vi "CAL_GCP_L_power.vi"(8 "L_power_raw":sgl, 9 "출력 클러스터 2":T1, 10 "B_ACC":sgl, 11 "L_ROLL":sgl) -> (0 "L_Period":sgl, 1 "L_GCP":sgl, 2 "L_Ctrl_Start":bool, 3 "L_NUM":u32, 4 "L_Run_OK":bool, 5 "출력 클러스터":T1)   [LabVIEW 2019]
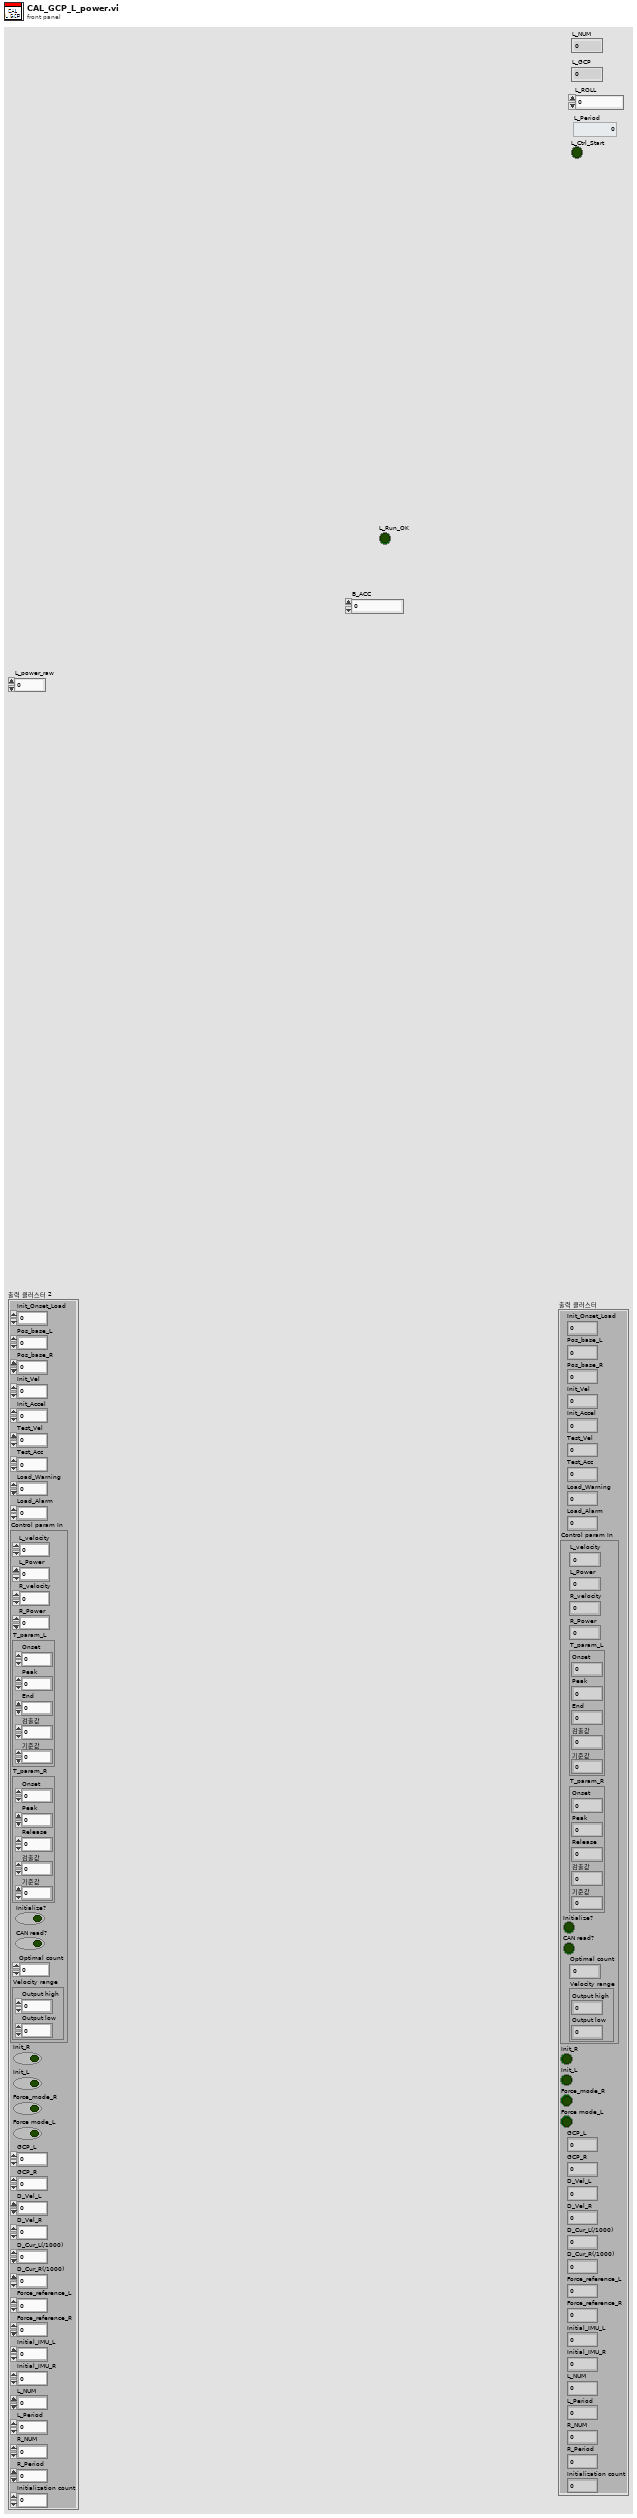
[diagram p1: front panel]
types:
  T1 = cluster{"Init_Onset_Load":sgl, "Pos_base_L":sgl, "Pos_base_R":sgl, "Init_Vel":i32, "Init_Accel":u32, "Test_Vel":i32, "Test_Acc":u32, "Load_Warning":sgl, "Load_Alarm":sgl, "Control param In":cluster{"L_velocity":u32, "L_Power":sgl, "R_velocity":u32, "R_Power":sgl, "T_param_L":cluster{"Onset":sgl, "Peak":sgl, "End":sgl, "검출값":sgl, "기준값":sgl}, "T_param_R":cluster{"Onset":sgl, "Peak":sgl, "Release":sgl, "검출값":sgl, "기준값":sgl}, "Initialize?":bool, "CAN read?":bool, "Optimal count":i32, "Velocity range":cluster{"Output high":dbl, "Output low":dbl}}, "Init_R":bool, "Init_L":bool, "Force_mode_R":bool, "Force mode_L":bool, "GCP_L":sgl, "GCP_R":sgl, "D_Vel_L":sgl, "D_Vel_R":sgl, "D_Cur_L(/1000)":sgl, "D_Cur_R(/1000)":sgl, "Force_reference_L":sgl, "Force_reference_R":sgl, "Initial_IMU_L":sgl, "Initial_IMU_R":sgl, "L_NUM":u32, "L_Period":i16, "R_NUM":u32, "R_Period":i16, "Initialization count":i32}
  T2 = enum16{"Init", "HF", "Cross", "HE", "Cross_E", "Init_F"}
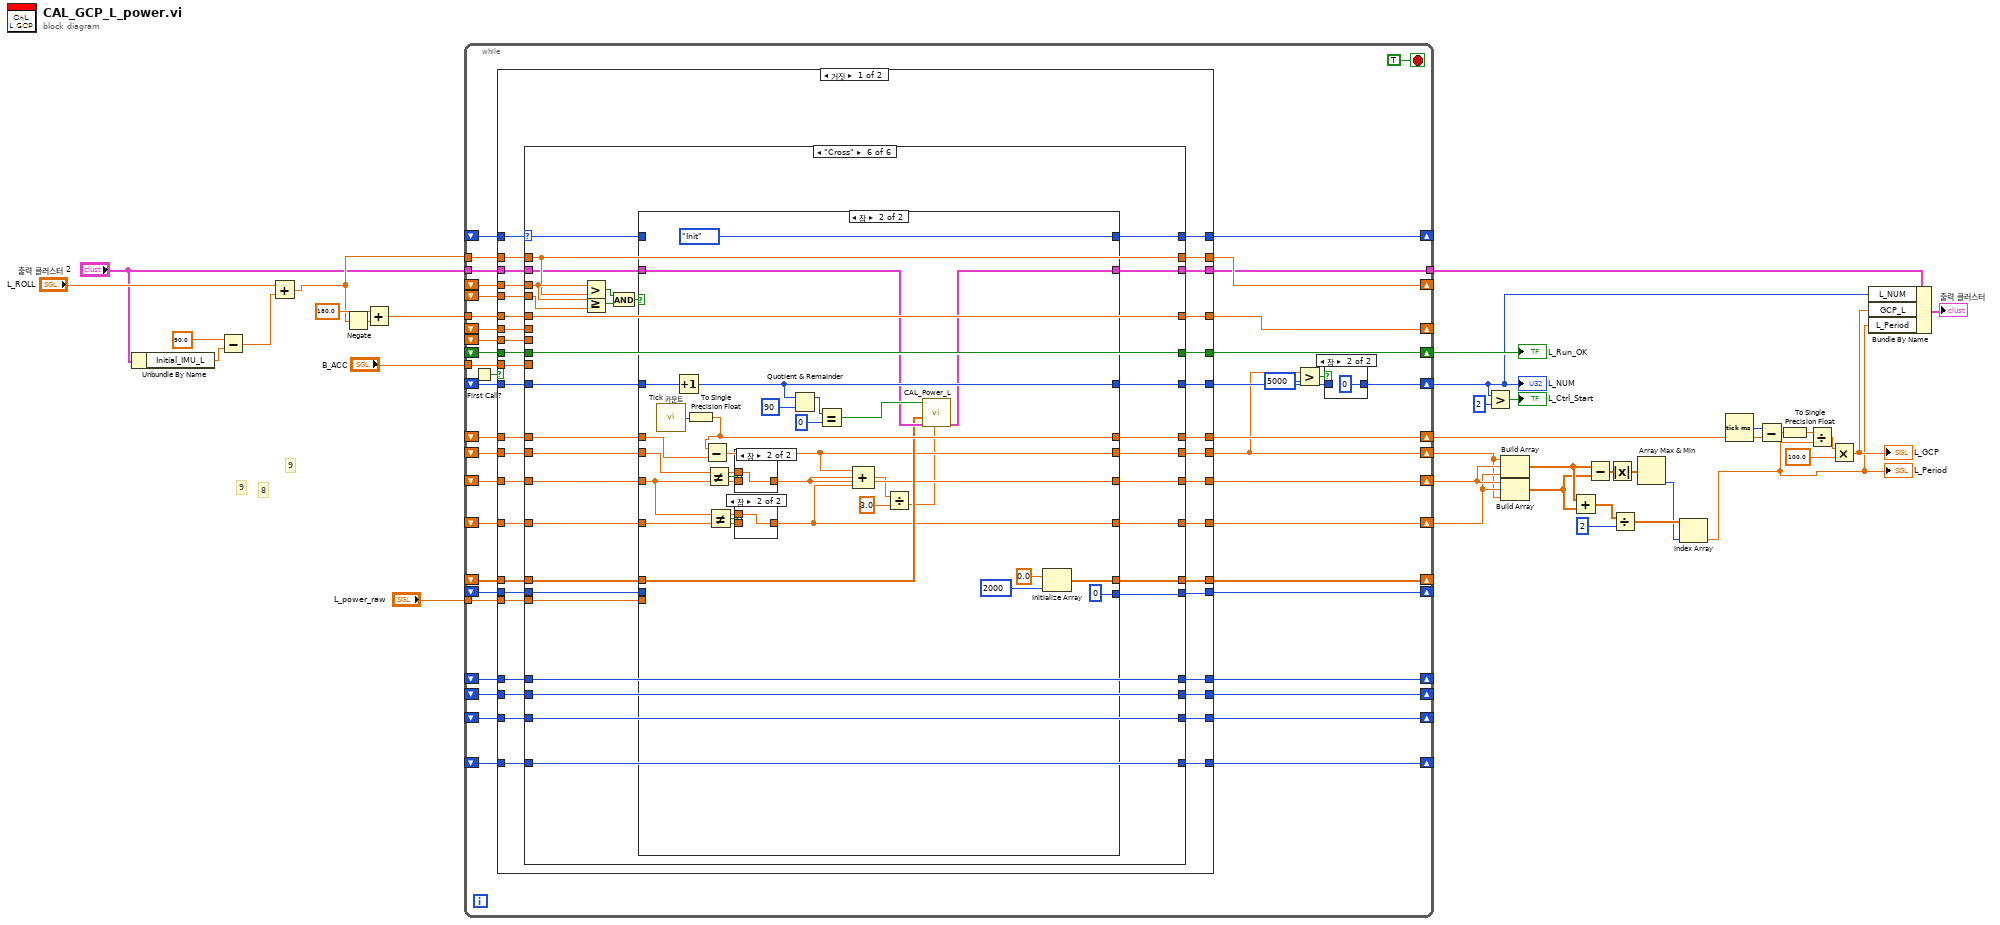
[diagram p0: block diagram]
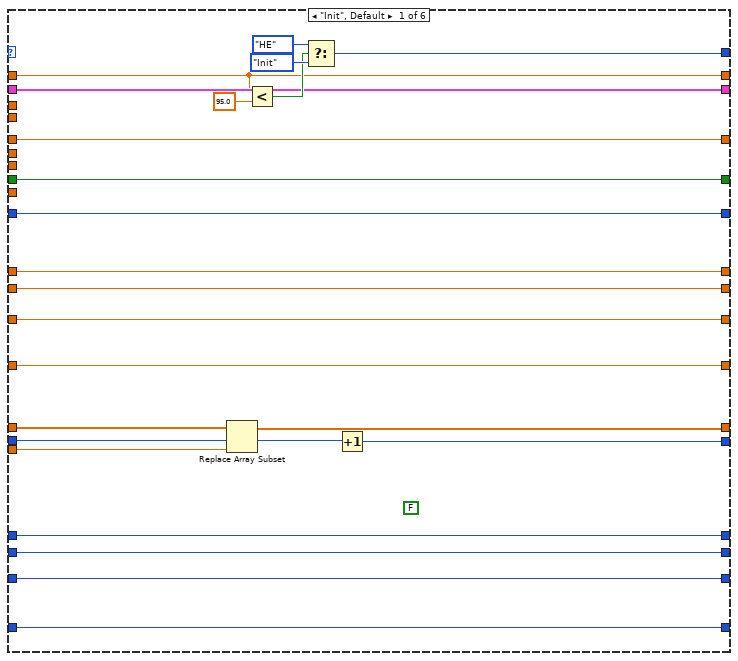
[diagram p2: hidden frame]
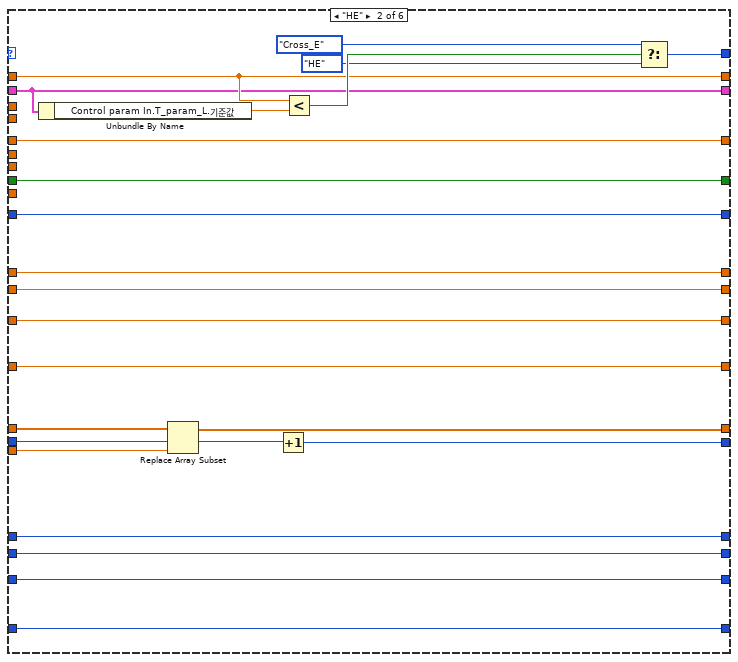
[diagram p3: hidden frame]
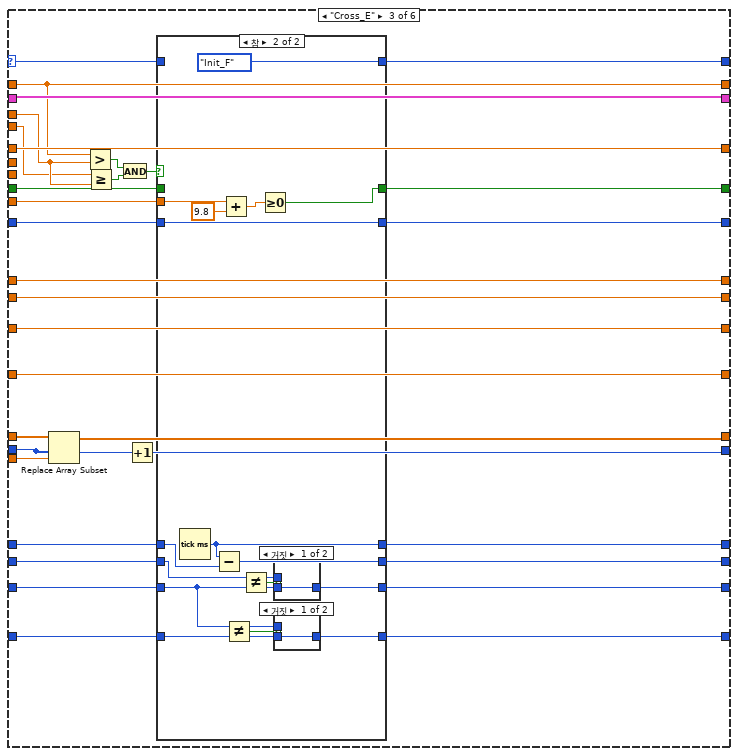
[diagram p4: hidden frame]
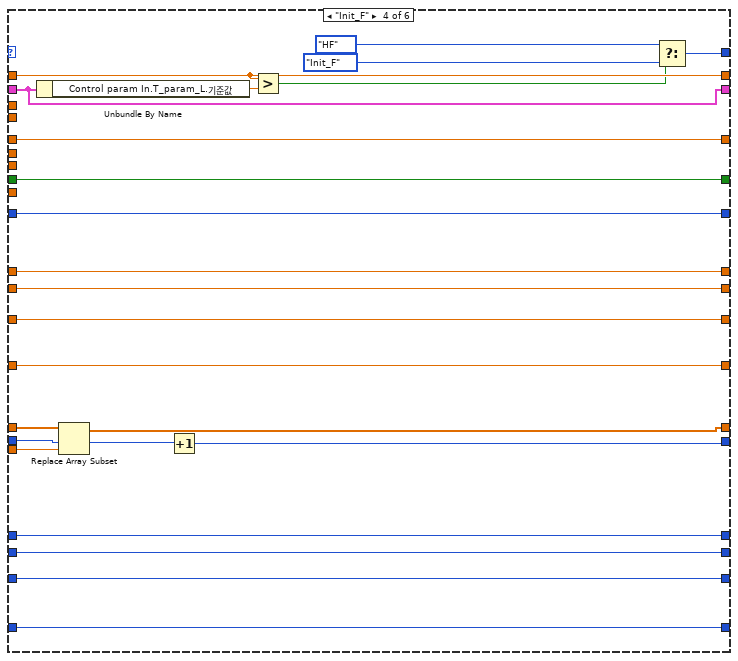
[diagram p8: hidden frame]
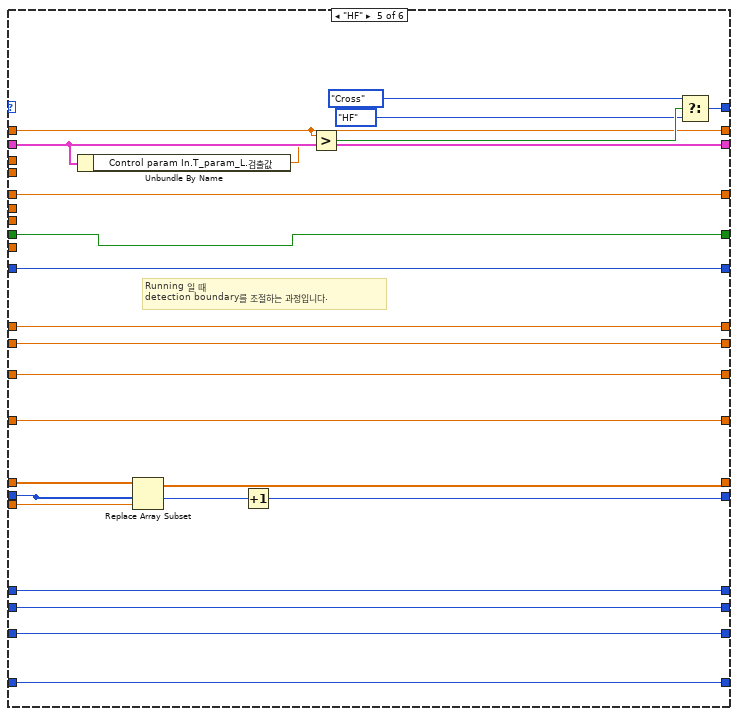
[diagram p9: hidden frame]
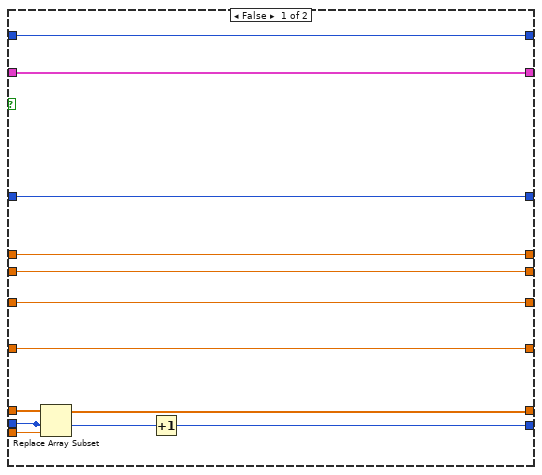
[diagram p10: hidden frame]
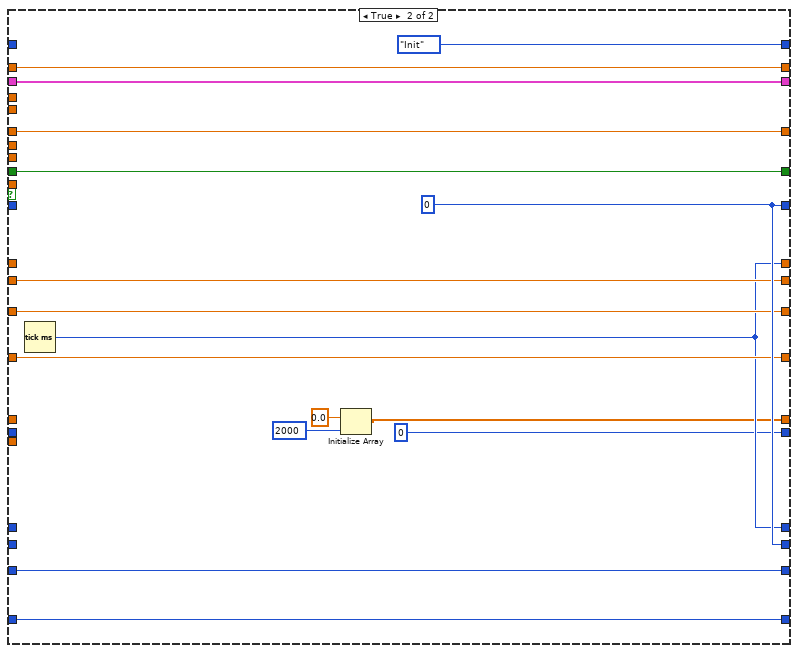
[diagram p13: hidden frame]
diagram:
  # "9"
  # "8"
  # "9"
  n1 = Unbundle By Name("출력 클러스터 2") -> ("Initial_IMU_L"=w5:sgl)
  n2 = Subtract(x=sgl 90.0 ("y"), y=w5) -> (x-y=w1:sgl)
  n3 = Add(x="L_ROLL", y=w1) -> (x+y=w12:sgl)
  n4 = Negate(x=w12) -> (-x=w28:sgl)
  n5 = Add(x=sgl 180.0, y=w28) -> (x+y=w27:sgl)
  n6 = while {
    tunnel: w12 -> [w76]
    tunnel: "출력 클러스터 2" -> [w73]
    shift-right: [w45] -> _
    shift-left: _ -> [w44]
    shift-right: [w77] -> _
    shift-left: _ -> [w72]
    shift-left: _ -> [w71]
    shift-right: [w68] -> w6
    shift-left: _ -> [w75]
    shift-right: [w58] -> _
    shift-left: _ -> [w74]
    tunnel: w27 -> [w66]
    shift-right: [w65] -> _
    shift-left: _ -> [w64]
    shift-left: _ -> [w63]
    shift-right: [w62] -> w25
    shift-left: _ -> [w61]
    tunnel: "B_ACC" -> [w60]
    shift-right: [w57] -> _
    shift-left: _ -> [w59]
    shift-right: [w50] -> w23
    shift-left: _ -> [w49]
    shift-right: [w47] -> w22
    shift-left: _ -> [w48]
    shift-right: [w56] -> _
    shift-left: _ -> [w55]
    shift-right: [w53] -> _
    shift-left: _ -> [w54]
    shift-right: [w52] -> w24
    shift-left: _ -> [w51]
    shift-right: [w43] -> w21
    shift-left: _ -> [w46]
    shift-right: [w42] -> _
    shift-left: _ -> [w40]
    tunnel: "L_power_raw" -> [w41]
    shift-right: [w39] -> _
    shift-left: _ -> [w38]
    tunnel: [w37] -> w9
    stop <- TRUE stop-if-true
    n7 = First Call?() -> (First Call?: T/F=w78:bool)
    n8 = case shown="거짓" w78 {
      tunnel: [w115 w359] -> w77
      tunnel: w76 -> [w116 w359]
      tunnel: w75 -> [w113 _]
      tunnel: [w114 w358] -> w67
      tunnel: [w111 w349] -> w58
      tunnel: [w110 w358] -> w57
      tunnel: w74 -> [w112 _]
      tunnel: w73 -> [w117 w344]
      tunnel: w72 -> [w109 _]
      tunnel: w71 -> [w108 _]
      tunnel: w66 -> [w107 w357]
      tunnel: [w106 w357] -> w65
      tunnel: w64 -> [w105 _]
      tunnel: w63 -> [w104 _]
      tunnel: [w102 w356] -> w62
      tunnel: w61 -> [w103 w356]
      tunnel: w60 -> [w101 _]
      tunnel: w59 -> [w100 _]
      tunnel: [w99 w355] -> w56
      tunnel: w55 -> [w98 w355]
      tunnel: w54 -> [w97 w354]
      tunnel: [w96 w354] -> w53
      tunnel: [w95 w349] -> w52
      tunnel: w51 -> [w94 _]
      tunnel: [w93 w353] -> w50
      tunnel: w49 -> [w92 w353]
      tunnel: w48 -> [w91 w352]
      tunnel: [w90 w352] -> w47
      tunnel: [w89 w351] -> w43
      tunnel: w46 -> [w88 w351]
      tunnel: [w86 T2."Init"] -> w45
      tunnel: w44 -> [w87 _]
      tunnel: [w85 w348] -> w42
      tunnel: w41 -> [w84 _]
      tunnel: w40 -> [w83 _]
      tunnel: [w81 0] -> w39
      tunnel: w38 -> [w82 _]
      tunnel: [w80 w344] -> w37
      frame False {
        n9 = case shown="\"Cross\"" w87 {
          selector: w87 -> [_ _ w195 _ _ w299]
          tunnel: w117 -> [w120 w142 w167 w223 w247 w270]
          tunnel: w116 -> [w119 w143 w166 w241 w267 w292]
          tunnel: [w119 w143 w166 w241 w267 w292] -> w115
          tunnel: [w140 w162 w193 w238 w266 w294] -> w114
          tunnel: w113 -> [w140 w162 w194 w238 w266 w295]
          tunnel: w112 -> [w139 w161 w191 w237 w265 w287]
          tunnel: [w139 w161 w192 w237 w265 w287] -> w111
          tunnel: [w136 w160 w190 w236 w264 w290] -> w110
          tunnel: w109 -> [_ _ w165 _ _ w293]
          tunnel: w108 -> [_ _ w164 _ _ w298]
          tunnel: w107 -> [w138 w156 w177 w240 w260 w284]
          tunnel: [w138 w156 w177 w240 w260 w284] -> w106
          tunnel: w105 -> [_ _ _ _ _ _]
          tunnel: w104 -> [_ _ _ _ _ _]
          tunnel: w103 -> [w137 w153 w189 w239 w257 w283]
          tunnel: [w137 w153 w188 w239 w257 w283] -> w102
          tunnel: w101 -> [_ _ w187 _ _ _]
          tunnel: w100 -> [w136 w160 w183 w236 w264 w290]
          tunnel: [w135 w159 w182 w234 w263 w289] -> w99
          tunnel: w98 -> [w135 w159 w181 w234 w263 w289]
          tunnel: w97 -> [w134 w158 w180 w233 w262 w288]
          tunnel: [w134 w158 w179 w233 w262 w288] -> w96
          tunnel: [w133 w157 w178 w235 w261 w286] -> w95
          tunnel: w94 -> [w133 w157 w178 w235 w261 w285]
          tunnel: [w132 w155 w175 w231 w259 w282] -> w93
          tunnel: w92 -> [w132 w155 w175 w231 w259 w281]
          tunnel: w91 -> [w131 w154 w176 w230 w258 w280]
          tunnel: [w131 w154 w176 w230 w258 w279] -> w90
          tunnel: [w130 w152 w174 w232 w256 w278] -> w89
          tunnel: w88 -> [w130 w152 w174 w232 w256 w277]
          tunnel: [w129 w149 w173 w242 w253 w276] -> w86
          tunnel: [w124 w145 w169 w225 w249 w275] -> w85
          tunnel: w84 -> [w121 w146 w170 w226 w250 w273]
          tunnel: w83 -> [w125 w148 w172 w228 w252 w274]
          tunnel: w82 -> [w123 w147 w171 w227 w251 w272]
          tunnel: [w122 w144 w168 w224 w248 w271] -> w81
          tunnel: [w120 w142 w167 w223 w247 w269] -> w80
          frame "Init", Default {
            (unwired) FALSE
            n10 = Replace Array Subset(array=w125, new element=w121, index=w123) -> (w124:sgl[])
            n11 = Less?(x=w119, y=sgl 95.0) -> (x < y?=w126:bool)
            n12 = Select(t=T2."HE", s=w126, f=T2."Init") -> (s? t:f=w129:T2)
            n13 = Increment(x=w123) -> (x+1=w122:i32)
          }
          frame "HE" {
            n14 = Unbundle By Name(w142) -> ("Control param In.T_param_L.기준값"=w141:sgl)
            n15 = Replace Array Subset(array=w148, new element=w146, index=w147) -> (w145:sgl[])
            n16 = Increment(x=w147) -> (x+1=w144:i32)
            n17 = Less?(x=w143, y=w141) -> (x < y?=w163:bool)
            n18 = Select(t=T2."Cross_E", s=w163, f=T2."HE") -> (s? t:f=w149:T2)
          }
          frame "Cross_E" {
            n19 = Replace Array Subset(array=w172, new element=w170, index=w171) -> (w169:sgl[])
            n20 = Greater?(x=w166, y=w165) -> (0:w185:bool)
            n21 = Greater Or Equal?(x=w164, y=w165) -> (x >= y?=w186:bool)
            n22 = And(x=w185, y=w186) -> (x .and. y?=w184:bool)
            n23 = Increment(x=w171) -> (x+1=w168:i32)
            n24 = case shown="참" w184 {
              tunnel: w195 -> [w200 _]
              tunnel: [w200 T2."Init_F"] -> w173
              tunnel: w194 -> [w201 w209]
              tunnel: [w201 w209] -> w193
              tunnel: w191 -> [w202 w218]
              tunnel: [w198 w208] -> w190
              tunnel: [w202 w217] -> w192
              tunnel: w189 -> [w199 _]
              tunnel: [w199 w214] -> w188
              tunnel: w187 -> [_ w205]
              tunnel: w183 -> [w198 w207]
              tunnel: [w197 w213] -> w182
              tunnel: w181 -> [w197 w206]
              tunnel: w180 -> [w196 w212]
              tunnel: [w196 w211] -> w179
              frame False {
              }
              frame True {
                n25 = Tick Count (ms)() -> (millisecond timer value=w217:u32)
                n26 = Subtract(x=w217, y=w218) -> (x-y=w208:u32)
                n27 = Add(x=w205, y=9.8) -> (x+y=w203:dbl)
                n28 = Not Equal?(x=w206, y=w212) -> (x != y?=w215:bool)
                n29 = Not Equal?(x=w207, y=w206) -> (x != y?=w216:bool)
                n30 = Greater Or Equal To 0?(x=w203) -> (x >= 0?=w214:bool)
                n31 = case shown="거짓" w216 {
                  tunnel: [w221 w222] -> w213
                  tunnel: w207 -> [_ w222]
                  tunnel: w206 -> [w221 _]
                  frame False {
                  }
                  frame True {
                  }
                }
                n32 = case shown="거짓" w215 {
                  tunnel: w206 -> [_ w220]
                  tunnel: w212 -> [w219 _]
                  tunnel: [w219 w220] -> w211
                  frame False {
                  }
                  frame True {
                  }
                }
              }
            }
          }
          frame "Init_F" {
            n33 = Unbundle By Name(w223) -> ("Control param In.T_param_L.기준값"=w245:sgl)
            n34 = Replace Array Subset(array=w228, new element=w226, index=w227) -> (w225:sgl[])
            n35 = Increment(x=w227) -> (x+1=w224:i32)
            n36 = Greater?(x=w241, y=w245) -> (0:w229:bool)
            n37 = Select(t=T2."HF", s=w229, f=T2."Init_F") -> (s? t:f=w242:T2)
          }
          frame "HF" {
            # "Running 일 때 \ndetection boundary를 조절하는 과정입니다."
            n38 = Unbundle By Name(w247) -> ("Control param In.T_param_L.검출값"=w246:sgl)
            n39 = Replace Array Subset(array=w252, new element=w250, index=w251) -> (w249:sgl[])
            n40 = Increment(x=w251) -> (x+1=w248:i32)
            n41 = Greater?(x=w267, y=w246) -> (0:w268:bool)
            n42 = Select(t=T2."Cross", s=w268, f=T2."HF") -> (s? t:f=w253:T2)
          }
          frame "Cross" {
            n43 = Greater?(x=w293, y=w292) -> (0:w291:bool)
            n44 = Greater Or Equal?(x=w293, y=w298) -> (x >= y?=w297:bool)
            n45 = And(x=w291, y=w297) -> (x .and. y?=w296:bool)
            n46 = case shown="참" w296 {
              tunnel: w299 -> [w310 _]
              tunnel: [w310 T2."Init"] -> w276
              tunnel: w295 -> [w311 w334]
              tunnel: [w311 w323] -> w294
              tunnel: [w309 w330] -> w286
              tunnel: w285 -> [w309 w337]
              tunnel: [w308 w317] -> w282
              tunnel: w281 -> [w308 w332]
              tunnel: w280 -> [w307 w336]
              tunnel: [w307 w316] -> w279
              tunnel: [w306 w318] -> w278
              tunnel: w277 -> [w306 w333]
              tunnel: [w302 w327] -> w275
              tunnel: w274 -> [w303 w319]
              tunnel: w273 -> [w304 _]
              tunnel: w272 -> [w305 _]
              tunnel: [w301 0] -> w271
              tunnel: w270 -> [w300 w321]
              tunnel: [w300 w320] -> w269
              frame False {
                n47 = Replace Array Subset(array=w303, new element=w304, index=w305) -> (w302:sgl[])
                n48 = Increment(x=w305) -> (x+1=w301:i32)
              }
              frame True {
                n49 = call "Tick 카운트"() -> ("Tick Count(mSec)"=w331:u32)
                n50 = Increment(x=w334) -> (x+1=w323:u32)
                n51 = To Single Precision Float(number=w331) -> (single precision float=w330:sgl)
                n52 = Subtract(x=w330, y=w337) -> (x-y=w318:sgl)
                n53 = Not Equal?(x=w333, y=w332) -> (x != y?=w339:bool)
                n54 = Not Equal?(x=w332, y=w336) -> (x != y?=w338:bool)
                n55 = case shown="참" w339 {
                  tunnel: w333 -> [_ w343]
                  tunnel: [w342 w343] -> w317
                  tunnel: w332 -> [w342 _]
                  frame False {
                  }
                  frame True {
                  }
                }
                n56 = case shown="참" w338 {
                  tunnel: w332 -> [_ w341]
                  tunnel: w336 -> [w340 _]
                  tunnel: [w340 w341] -> w316
                  frame False {
                  }
                  frame True {
                  }
                }
                n57 = Quotient & Remainder(x=w323, y=u32 90) -> (x-y*floor(x/y)=w325:u32)  [unwired: 1 out]
                n58 = Equal?(x=w325, y=u32 0) -> (x = y?=w322:bool)
                n59 = Compound Arithmetic op=ADD(w318, w317, w316) -> (w315:sgl)
                n60 = Divide(x=w315, y=sgl 3.0) -> (x/y=w313:sgl)
                n61 = call "CAL_Power_L.vi"("stride?"=w322, "Positive Power"=w319, "출력 클러스터 2"=w321, "Period_L"=w313) -> ("출력 클러스터 3"=w320:T1)  [unwired: 6 in]
                n62 = Initialize Array(sgl 0.0 ("원소"), 2000 ("차원 크기")) -> (w327:sgl[])
              }
            }
          }
        }
      }
      frame True {
        w358 = u32 0
        n63 = Tick Count (ms)() -> (millisecond timer value=w349:u32)
        n64 = Initialize Array(sgl 0.0 ("원소"), 2000 ("차원 크기")) -> (w348:sgl[])
      }
    }
    n65 = Greater?(x=w43, y=u32 5000) -> (0:w69:bool)
    n66 = case shown="참" w69 {
      tunnel: [w360 u32 0] -> w68
      tunnel: w67 -> [w360 _]
      frame False {
      }
      frame True {
      }
    }
  }
  "L_NUM" <- w6
  "L_Run_OK" <- w25
  n67 = Greater?(x=w6, y=u32 2) -> (0:→"L_Ctrl_Start":bool)
  n68 = Build Array(w21, w23, w22) -> (w14:sgl[])
  n69 = Build Array(w23, w22, w21) -> (w13:sgl[])
  n70 = Add(x=w14, y=w13) -> (x+y=w18:sgl[])
  n71 = Subtract ("빼기")(x=w14, y=w13) -> (x-y=w20:sgl[])
  n72 = Absolute Value(x=w20) -> (abs(x)=w19:sgl[])
  n73 = Divide ("나누기")(x=w18, y=2) -> (x/y=w16:sgl[])
  n74 = Array Max & Min(array=w19) -> (min index (indices)=w15:i32)  [unwired: 3 out]
  n75 = Index Array(array=w16, index=w15) -> (element=w7:sgl)
  "L_Period" <- w7
  n76 = Tick Count (ms)() -> (millisecond timer value=w32:u32)
  n77 = Subtract(x=w32, y=w24) -> (x-y=w31:sgl)
  n78 = To Single Precision Float(number=w31) -> (single precision float=w30:sgl)
  n79 = Divide(x=w30, y=w7) -> (x/y=w34:sgl)
  n80 = Multiply(x=w34, y=sgl 100.0) -> (x*y=w8:sgl)
  "L_GCP" <- w8
  n81 = Bundle By Name(cluster=w9, "L_NUM"=w6, "GCP_L"=w8, "L_Period"=w7) -> (→"출력 클러스터":T1)
